vi "CoincidenceHistogram.vi"(1 "coincidence histogram in":T1={"origin (ns)"=0.0, "offset (ns)"=100.0, "histogram"=[]} {"offset (ns)" format="%.2f"; "origin (ns)" format="%.2f"}, 2 "set":bool) -> (0 "coincidence histogram out":T1={"origin (ns)"=0.0, "offset (ns)"=100.0, "histogram"=[]} {"offset (ns)" format="%.2f"; "origin (ns)" format="%.2f"})   [LabVIEW 2009]
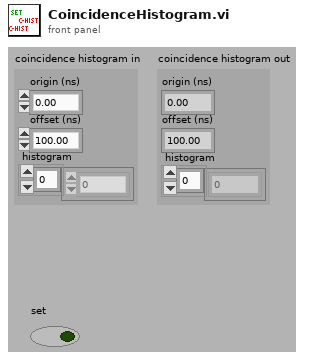
[diagram p1: front panel]
types:
  T1 = cluster{"origin (ns)":dbl, "offset (ns)":dbl, "histogram":u32[]}
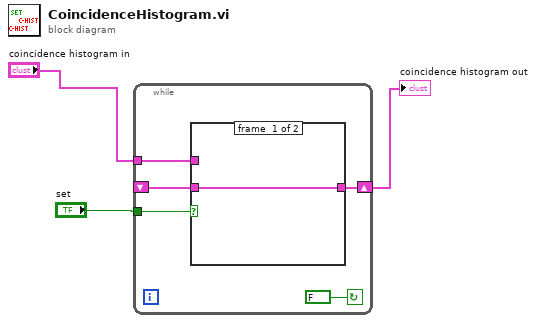
[diagram p0: block diagram]
diagram:
  n1 = while {
    shift-right: [w6] -> w1
    shift-left: _ -> [w4]
    tunnel: "set" -> [w7]
    tunnel: "coincidence histogram in" -> [w5]
    stop <- FALSE continue-if-true
    n2 = case shown="True" w7 {
      tunnel: [w9 w10] -> w6
      tunnel: w5 -> [_ w10]
      tunnel: w4 -> [w9 _]
      frame #0 {
      }
      frame #1 {
      }
    }
  }
  "coincidence histogram out" <- w1
